vi "GetFileList.vi"(8 "pattern":string, 9 "HighSpeedEServer":refnum<k24>, 11 "error in (no error)":errorcluster) -> (1 "Files":string[](array[string]), 3 "error out":errorcluster)   [LabVIEW 2020, in "UnderAutomation.Yaskawa.lvlib"]
uses:
  UnderAutomation.Yaskawa.lvlib
  C:/Users/fg/Documents/Yaskawa.vi/LabVIEW_2024/UnderAutomation.Yaskawa/lib/UnderAutomation.Yaskawa.dll
  LabVIEW_2024/UnderAutomation.Yaskawa/lib/UnderAutomation.Yaskawa.dll
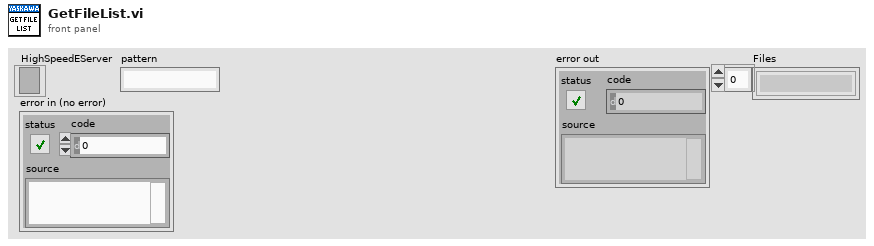
[diagram p1: front panel]
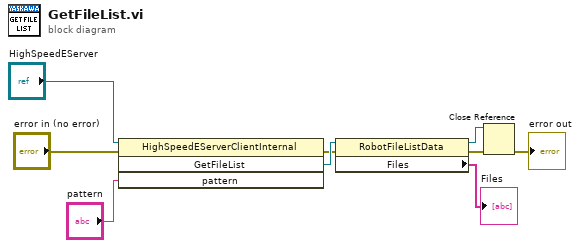
[diagram p0: block diagram]
diagram:
  n1 = invoke class="HighSpeedEServerClientInternal" method="GetFileList"(reference="HighSpeedEServer", error in="error in (no error)", "pattern"="pattern") -> (error out=w5:errorcluster, "GetFileList"=w6:refnum<k24>)  [unwired: 1 in, 2 out]
  n2 = property class="RobotFileListData"(reference=w6, error in=w5) -> (reference out=w1:refnum<k24>, error out=w3:errorcluster, "Files"=→"Files":string[])
  n3 = Close Reference(reference=w1, error in (no error)=w3) -> (error out=→"error out":errorcluster)
